vi "DB HOR count.vi"(0 "file path":path, 13 "gap":i32) -> (8 "number of scans":i32)   [LabVIEW 2014]
panel:
  # "Calculates the total number of files to read\ntaking in to account the gap between files"
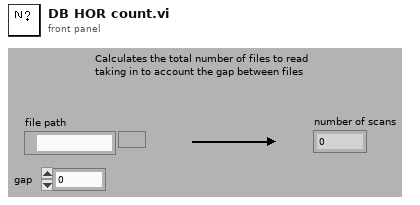
[diagram p1: front panel]
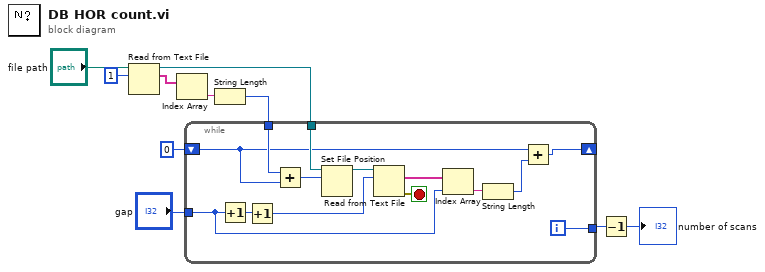
[diagram p0: block diagram]
diagram:
  n1 = Read from Text File(file (use dialog)="file path", count=1) -> (refnum out=w6:refnum<file>, text=w8:string[])  [unwired: 2 in, 2 out]
  n2 = Index Array(array=w8) -> (element=w7:string)  [unwired: 1 in]
  n3 = String Length(string=w7) -> (length=w5:i32)
  n4 = while {
    tunnel: w6 -> [w21]
    tunnel: w5 -> [w19]
    tunnel: "gap" -> [w13]
    shift-right: [w11] -> _
    shift-left: 0 -> [w18]
    tunnel: [w14] -> w3
    i -> [w14]
    stop <- w15 stop-if-true
    n5 = Increment(x=w13) -> (x+1=w12:i32)
    n6 = Increment(x=w12) -> (x+1=w16:i32)
    n7 = Add(x=w19, y=w18) -> (x+y=w20:i32)
    n8 = Set File Position(offset (in bytes) (0)=w20, refnum=w21) -> (refnum out=w24:refnum<file>)  [unwired: 2 in, 1 out]
    n9 = Read from Text File(file (use dialog)=w24, count=w16) -> (text=w22:string[], error out=w15:errorcluster)  [unwired: 2 in, 2 out]
    n10 = Index Array(array=w22, index=w13) -> (element=w23:string)
    n11 = String Length(string=w23) -> (length=w17:i32)
    n12 = Add(x=w18, y=w17) -> (x+y=w11:i32)
  }
  n13 = Decrement(x=w3) -> (x-1=→"number of scans":i32)
